vi "Read Mfg Test Timestamp.vi"(8 "error in":errorcluster) -> (0 "error out":errorcluster, 3 "time stamp":timestamp)   [LabVIEW 2015]
uses:
  CAN Communication/Gas/Gas.lvclass
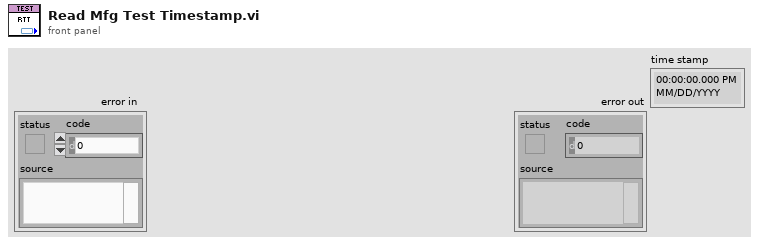
[diagram p1: front panel]
types:
  T1 = typedef "Gas.lvclass/Session Handle.ctl" = refnum<data-value>
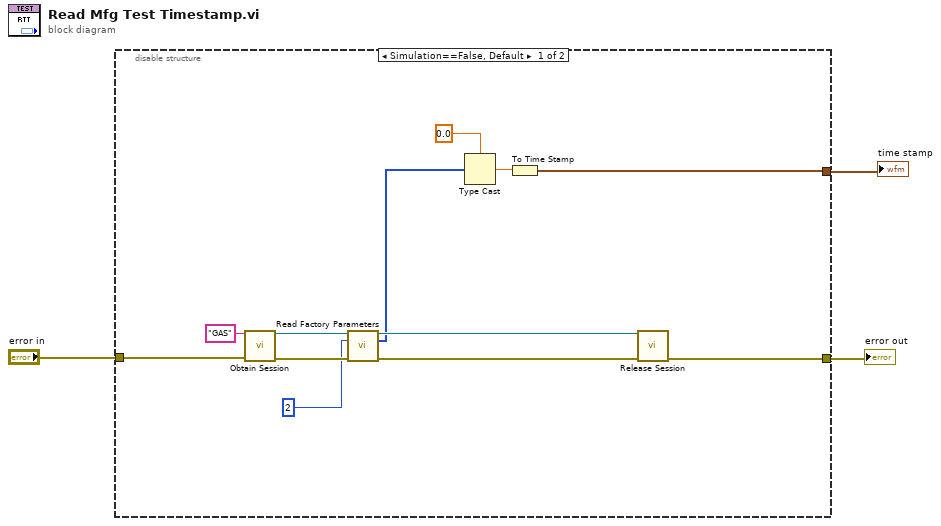
[diagram p0: block diagram]
diagram:
  n1 = disable-structure shown="Simulation==False, Default" {
    disable-tunnel: [w11 w16] -> w3
    disable-tunnel: "error in" -> [w10 w16]
    disable-tunnel: [w4 _] -> w1
    frame condition #0 (active) {
      n2 = call "Obtain Session.vi"("Session  Name ()"="GAS", "error in (no error)"=w10) -> ("Session Handle"=w15:T1, "error out"=w14:errorcluster)  [unwired: 12 in]
      n3 = call "Read Factory Parameters.vi"("Session Handle in"=w15, "Address"=2, "error in (no error)"=w14) -> ("Session Handle out"=w13:T1, "Read Bytes"=w7:u8[], "error out"=w12:errorcluster)  [unwired: 10 in]
      n4 = Type Cast(type=sgl 0.0, x=w7) -> (*(type *) &x=w5:sgl)
      n5 = To Time Stamp(1:w5) -> (0:w4:timestamp)
      n6 = call "Release Session.vi"("Session Handle"=w13, "error in (no error)"=w12) -> ("error out"=w11:errorcluster)  [unwired: 13 in]
    }
    frame condition #1 {
    }
  }
  "error out" <- w3
  "time stamp" <- w1
